vi "Fetch gRPC Server from Map.vi"(7 "gRPC Server Class type":refnum<class "PluginCore.lvclass">, 8 "error in (no error)":errorcluster, 11 "CIFCorePlugin in":refnum<class "CIFCorePlugin.lvclass">) -> (0 "error out":errorcluster, 2 "gRPC Server Class out":refnum<class "PluginCore.lvclass">, 3 "CIFCorePlugin out":refnum<class "CIFCorePlugin.lvclass">)   [LabVIEW 2021, in "CIFCorePlugin.lvclass"]
uses:
  CIFCorePlugin.lvclass
  CIFCorePlugin.lvclass/CIFCorePlugin.ctl
  Typedef/Error Global.vi
  CIFCoreGrpc/CIFCorePlugin_server/RPC Service/PluginCore/PluginCore.lvclass
  C:/Program Files/National Instruments/LabVIEW 2021/vi.lib/gRPC/LabVIEW gRPC Servicer/ServiceBase/ServiceBase.lvclass
  D:/dev/CIF-LVCore/src/CIFCore/CIFCoreGrpc/CIFCorePlugin_server/RPC Service/PluginCore/PluginCore.lvclass
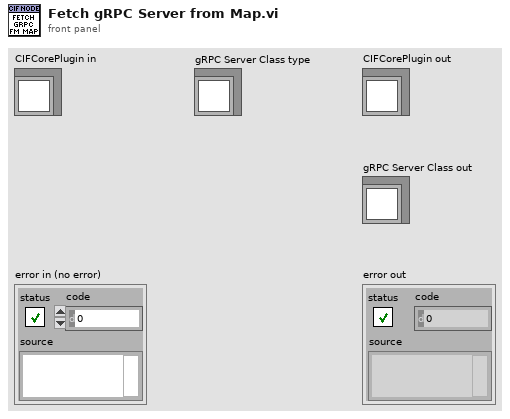
[diagram p1: front panel]
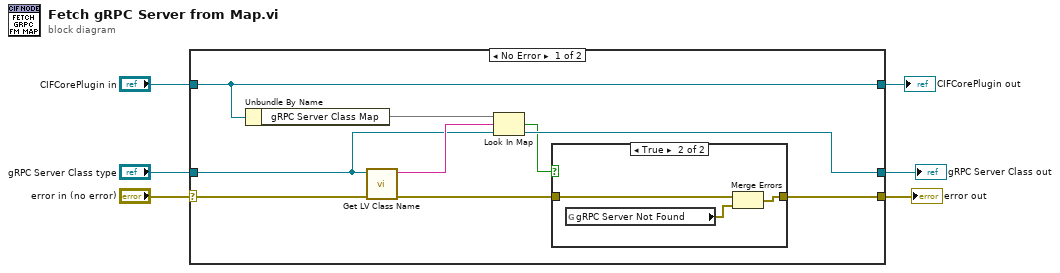
[diagram p0: block diagram]
diagram:
  n1 = case shown="No Error" "error in (no error)" {
    selector: "error in (no error)" -> [w14 w21]
    tunnel: [w7 w21] -> w5
    tunnel: [w15 w22] -> w3
    tunnel: "CIFCorePlugin in" -> [w15 w22]
    tunnel: "gRPC Server Class type" -> [w10 w20]
    tunnel: [w11 w20] -> w1
    frame No Error {
      n2 = Unbundle By Name(w15) -> ("gRPC Server Class Map"=w12:map{string, refnum<class "PluginCore.lvclass">})
      n3 = call <vilib>:"Get LV Class Name.vi"("error in (no error)"=w14, "object"=w10) -> ("error out"=w8:errorcluster, "class name"=w13:string)  [unwired: 8 in]
      n4 = Look In Map(map=w12, key=w13, default value=w10) -> (key not found?=w9:bool, value=w11:refnum<class "PluginCore.lvclass">)
      n5 = case shown="True" w9 {
        tunnel: w8 -> [w16 w19]
        tunnel: [w16 w17] -> w7
        frame False {
        }
        frame True {
          n6 = global read "Error Global.vi" "gRPC Server Not Found"() -> (w18:errorcluster)
          n7 = Merge Errors(w19, w18) -> (w17:errorcluster)
        }
      }
    }
    frame Error {
    }
  }
  "error out" <- w5
  "CIFCorePlugin out" <- w3
  "gRPC Server Class out" <- w1
